vi "FL_DEC_split_3_and_prefilter.vi"(0 "DEC input cluster":T4, 1 "Pre-filter params.":T1, 2 "Initialize? (F)":bool) -> (3 "Times":T3, 4 "TTLs":cluster{"TTL in 1":i16, "TTL in 2":i16}, 5 "Magnets coords":cluster{"X1":dbl, "Y1":dbl, "X2":dbl, "Y2":dbl}, 6 "Magnets coords raw":T2)   [LabVIEW 2018, in "Tracker.lvlib"]
uses:
  Tracker.lvlib
  Controls/CTL_Decoded_data_frame.ctl
  Controls/CTL_Pre-filter_params.ctl
  <vilib>/ptbypt/NI_PtbyPt.lvlib
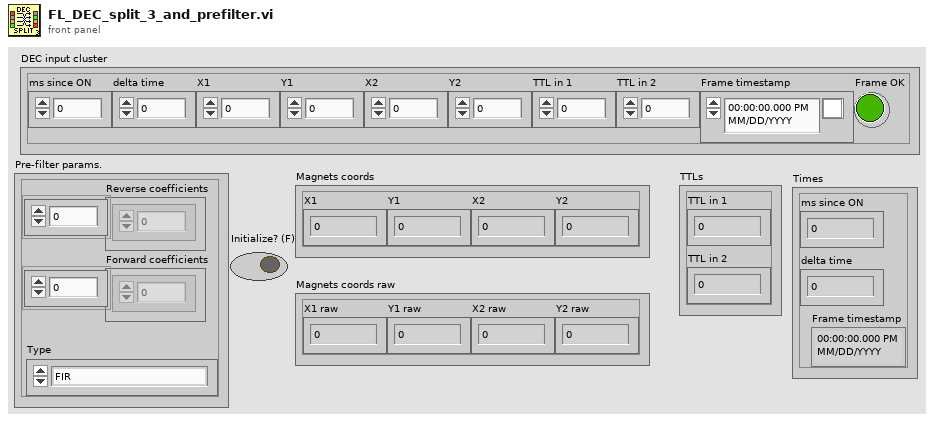
[diagram p1: front panel]
types:
  T1 = typedef "Tracker.lvlib/CTL_Pre-filter_params.ctl" = cluster{"Reverse coefficients":dbl[], "Forward coefficients":dbl[], "Type":enum16{"FIR", "IIR"}}
  T2 = cluster{"X1 raw":dbl, "Y1 raw":dbl, "X2 raw":dbl, "Y2 raw":dbl}
  T3 = cluster{"ms since ON":u32, "delta time":u32, "Frame timestamp":timestamp}
  T4 = typedef "Tracker.lvlib/CTL_Decoded_data_frame.ctl" = cluster{"ms since ON":u32, "delta time":u32, "X1":sgl, "Y1":sgl, "X2":sgl, "Y2":sgl, "TTL in 1":i16, "TTL in 2":i16, "Frame timestamp":timestamp, "Frame OK":bool}
  T5 = cluster{"Filtered x":dbl, "Filtered x":dbl, "Filtered x":dbl, "Filtered x":dbl}
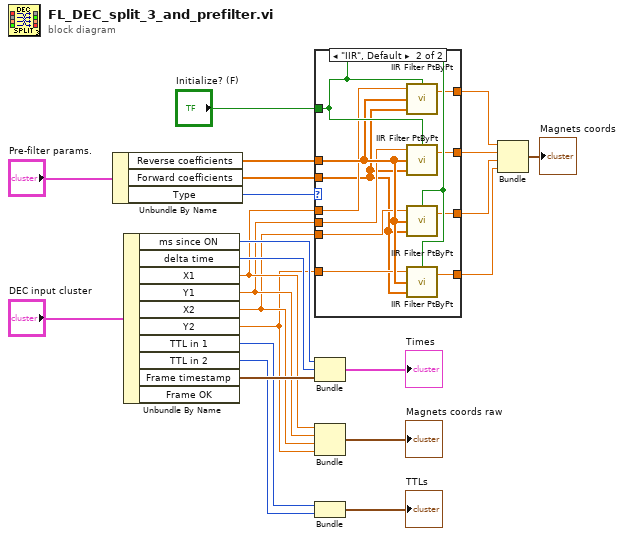
[diagram p0: block diagram]
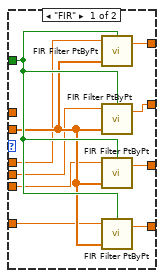
[diagram p2: hidden frame]
diagram:
  n1 = Unbundle By Name("Pre-filter params.") -> ("Reverse coefficients"=w12:dbl[], "Forward coefficients"=w11:dbl[], "Type"=w13:enum16{"FIR", "IIR"})
  n2 = Unbundle By Name("DEC input cluster") -> ("ms since ON"=w22:u32, "delta time"=w21:u32, "X1"=w9:sgl, "Y1"=w8:sgl, "X2"=w7:sgl, "Y2"=w6:sgl, "TTL in 1"=w18:i16, "TTL in 2"=w17:i16, "Frame timestamp"=w20:timestamp)  [unwired: 1 out]
  n3 = case shown="\"IIR\", Default" w13 {
    tunnel: w12 -> [_ w43]
    tunnel: w11 -> [w32 w34]
    tunnel: "Initialize? (F)" -> [w33 w44]
    tunnel: w9 -> [w31 w42]
    tunnel: w8 -> [w29 w41]
    tunnel: w7 -> [w27 w40]
    tunnel: w6 -> [w25 w39]
    tunnel: [w30 w38] -> w5
    tunnel: [w28 w37] -> w4
    tunnel: [w26 w36] -> w3
    tunnel: [w24 w35] -> w2
    frame "FIR" {
      n4 = call <vilib>:"FIR Filter PtByPt.vi"("initialize"=w33, "Forward Coefficients"=w32, "x"=w31) -> ("Filtered x"=w30:dbl)  [unwired: 1 in, 1 out]
      n5 = call <vilib>:"FIR Filter PtByPt.vi"("initialize"=w33, "Forward Coefficients"=w32, "x"=w29) -> ("Filtered x"=w28:dbl)  [unwired: 1 in, 1 out]
      n6 = call <vilib>:"FIR Filter PtByPt.vi"("initialize"=w33, "Forward Coefficients"=w32, "x"=w27) -> ("Filtered x"=w26:dbl)  [unwired: 1 in, 1 out]
      n7 = call <vilib>:"FIR Filter PtByPt.vi"("initialize"=w33, "Forward Coefficients"=w32, "x"=w25) -> ("Filtered x"=w24:dbl)  [unwired: 1 in, 1 out]
    }
    frame "IIR", Default {
      n8 = call <vilib>:"IIR Filter PtByPt.vi"("initialize"=w44, "Forward Coefficients"=w34, "Reverse Coefficients"=w43, "x"=w42) -> ("Filtered x"=w38:dbl)  [unwired: 1 out]
      n9 = call <vilib>:"IIR Filter PtByPt.vi"("initialize"=w44, "Forward Coefficients"=w34, "Reverse Coefficients"=w43, "x"=w41) -> ("Filtered x"=w37:dbl)  [unwired: 1 out]
      n10 = call <vilib>:"IIR Filter PtByPt.vi"("initialize"=w44, "Forward Coefficients"=w34, "Reverse Coefficients"=w43, "x"=w40) -> ("Filtered x"=w36:dbl)  [unwired: 1 out]
      n11 = call <vilib>:"IIR Filter PtByPt.vi"("initialize"=w44, "Forward Coefficients"=w34, "Reverse Coefficients"=w43, "x"=w39) -> ("Filtered x"=w35:dbl)  [unwired: 1 out]
    }
  }
  n12 = Bundle("ms since ON"=w22, "delta time"=w21, "Frame timestamp"=w20) -> (→"Times":T3)  [unwired: 1 in]
  n13 = Bundle("X1"=w9, "Y1"=w8, "X2"=w7, "Y2"=w6) -> (→"Magnets coords raw":cluster{"X1":sgl, "Y1":sgl, "X2":sgl, "Y2":sgl})  [unwired: 1 in]
  n14 = Bundle("TTL in 1"=w18, "TTL in 2"=w17) -> (→"TTLs":cluster{"TTL in 1":i16, "TTL in 2":i16})  [unwired: 1 in]
  n15 = Bundle("Filtered x"=w5, "Filtered x"=w4, "Filtered x"=w3, "Filtered x"=w2) -> (→"Magnets coords":T5)  [unwired: 1 in]
